vi "Application (WIP).vi"() -> ()   [LabVIEW 2018, in "Application.lvlib"]
uses:
  Application.lvlib
  Potentiostat Galvanostat Class/Controls/CV Parameters.ctl
  Potentiostat Galvanostat Class/Controls/OCV Parameters.ctl
  Potentiostat Galvanostat Class/Controls/CA Parameters.ctl
  Potentiostat Galvanostat Class/Controls/CP Parameters.ctl
  Potentiostat Galvanostat Class/Controls/PEIS Parameters.ctl
  Potentiostat Galvanostat Class/Controls/GEIS Parameters.ctl
  Potentiostat Galvanostat Class/Potentiostat Galvanostat.lvclass
panel:
  in  "DLL Path":path=path "C:/EC-Lab Development Package/EC-Lab Development Package/EClib.dll"
  out "Connected?":bool
  in  "Timeout":dbl=5.0 format="%#_g s"
  in  "IP Address/USB":string="192.109.209.128"
  in  "Disconnect":bool
  in  "Connect":bool
  out "Number of Connected PCs":i32
  out "Number of Slots":i32
  out "Number of Channels":i32
  out "Firmware Date":string
  out "Firmware Version":i32
  out "Device Code":string
  in  "Graph":bool
  in  "Stop":bool
  in  "Start":bool
  in  "Technique Parameters Tab":enum32{"ocv", "cv", "ca", "cp", "peis", "geis"}(tab)=enum."cv" caption="Parameters"
  in  "OCV Parameters":T1={"Rest duration (s)"=1.0, "Record every dE (V)"=0.01, "Record every dT (s)"=0.01, "Ewe range"=3, "CE to ground Mode"=0} {"Ewe range" items=["±2.5V", "±5V", "±10V", "Auto"]; "Record every dT (s)" min=0 format="%.2e"; "Record every dE (V)" min=0 max=100 format="%.4f"; "Rest duration (s)" min=0 format="%.2f"; "CE to ground Mode" items=["Standard", "CE to ground"]}
  in  "CV Parameters":T2={"Ei Params"={"Current step vs initial one (Ei)"=TRUE, "Voltage step (V) (Ei)"=0.0, "slew rate array (mV/s) (Ei)"=0.1}, "E1 Params"={"Current step vs initial one (E1)"=FALSE, "Voltage step (V) (E1)"=0.1, "slew rate array (mV/s) (E1)"=0.1}, "E2 Params"={"Current step vs initial one (E2)"=FALSE, "Voltage step (V) (E2)"=-0.2, "slew rate array (mV/s) (E2)"=0.1}, "Ef Params"={"Current step vs initial one (Ef)"=TRUE, "Voltage step (V) (Ef)"=0.0, "slew rate array (mV/s) (Ef)"=0.1}, "Number of cycle"=1, "recording on dE (V)"=0.01, "average every dE"=TRUE, "Begin step accumulation (1 = 100% of step)"=0.5, "End step accumulation ( 1 = 100% of step)"=0.75, "I range"=12, "Bandwidth"=5, "Ewe range"=3, "CE to ground Mode"=0} {"CE to ground Mode" items=["Standard", "CE to ground"]; "Ewe range" items=["±2.5V", "±5V", "±10V", "Auto"]; "Bandwidth" items=["1 - slow"=1, "2"=2, "3"=3, "4"=4, "5 - medium"=5, "6"=6, "7 - fast"=7]; "I range" items=["1pA", "1nA", "10nA", "100nA", "1µA", "10µA", "100µA", "1mA", "10mA", "100mA", "1A", "Booster", "Auto"]; "End step accumulation ( 1 = 100% of step)" min=0 max=1 format="%_2f"; "Begin step accumulation (1 = 100% of step)" min=0 max=1 format="%_2f"; "recording on dE (V)" min=0 max=100 format="%^_3e"; "Number of cycle" min=0 max=1000000; "Ef Params"."slew rate array (mV/s) (Ef)" min=1e-07 max=100000 format="%_5e"; "Ef Params"."Voltage step (V) (Ef)" min=-10 max=10 format="%_5e"; "E2 Params"."slew rate array (mV/s) (E2)" min=1e-07 max=100000 format="%_5e"; "E2 Params"."Voltage step (V) (E2)" min=-10 max=10 format="%_5e"; "E1 Params"."slew rate array (mV/s) (E1)" min=1e-07 max=100000 format="%_5e"; "E1 Params"."Voltage step (V) (E1)" min=-10 max=10 format="%_5e"; "Ei Params"."slew rate array (mV/s) (Ei)" min=1e-07 max=100000 format="%_5e"; "Ei Params"."Voltage step (V) (Ei)" min=-10 max=10 format="%_5e"}
  in  "CA Parameters":T3={"Voltage Steps"=[{"Voltage step vs initial one"=TRUE, "Voltage step (V)"=0.0, "Duration step (s)"=1.0}, {"Voltage step vs initial one"=TRUE, "Voltage step (V)"=0.1, "Duration step (s)"=1.0}, {"Voltage step vs initial one"=TRUE, "Voltage step (V)"=0.2, "Duration step (s)"=1.0}], "No. of steps"=2, "Record every dt (s)"=0.01, "Record every dI (A)"=1e-05, "No. of times\ntechnique is repeated"=0, "I range"=12, "Ewe range"=3, "Bandwidth"=5, "CE to ground Mode"=0} {"Voltage Steps"."Duration step (s)" min=0.001 max=80000 format="%^_3e"; "Voltage Steps"."Voltage step (V)" min=-10 max=10 format="%^_3e"; "No. of times\ntechnique is repeated" min=0 max=1000000; "No. of steps" min=0 max=99; "Record every dt (s)" min=0.0001 max=1000 format="%^_3e"; "Record every dI (A)" format="%^_3e"; "CE to ground Mode" items=["Standard", "CE to ground"]; "Ewe range" items=["±2.5V", "±5V", "±10V", "Auto"]; "Bandwidth" items=["1 - slow"=1, "2"=2, "3"=3, "4"=4, "5 - medium"=5, "6"=6, "7 - fast"=7]; "I range" items=["1pA", "1nA", "10nA", "100nA", "1µA", "10µA", "100µA", "1mA", "10mA", "100mA", "1A", "Booster", "Auto"]}
  in  "CP Parameters":T4={"Current Steps"=[{"Current step vs initial\none"=FALSE, "Current step (A)"=0.0, "Duration step (s)"=1.0}, {"Current step vs initial\none"=FALSE, "Current step (A)"=0.001, "Duration step (s)"=1.0}, {"Current step vs initial\none"=FALSE, "Current step (A)"=0.005, "Duration step (s)"=1.0}], "No. of steps"=2, "Record every dt (s)"=0.05, "Record every dE (V)"=0.005, "No. of times\ntechnique is repeated"=0, "I range"=8, "Ewe range"=3, "Bandwidth"=5, "CE to ground Mode"=0} {"Current Steps"."Duration step (s)" min=0.001 max=80000 format="%^_3e"; "Current Steps"."Current step (A)" min=-150 max=150 format="%^_3e"; "No. of times\ntechnique is repeated" min=0 max=1000000; "No. of steps" min=0 max=99; "Record every dt (s)" min=0.0001 max=1000 format="%^_3e"; "Record every dE (V)" format="%^_3e"; "CE to ground Mode" items=["Standard", "CE to ground"]; "Ewe range" items=["±2.5V", "±5V", "±10V", "Auto"]; "Bandwidth" items=["1 - slow"=1, "2"=2, "3"=3, "4"=4, "5 - medium"=5, "6"=6, "7 - fast"=7]; "I range" items=["1pA", "1nA", "10nA", "100nA", "1µA", "10µA", "100µA", "1mA", "10mA", "100mA", "1A", "Booster", "Auto"]}
  in  "PEIS Parameters":T5={"Step duration (s)"=1.0, "Record every dI (A)"=0.1, "Record every dt (s)"=0.1, "Initial voltage step (V)"=0.0, "Voltage step vs initial one"=TRUE, "Initial frequency (Hz)"=100000.0, "sweep linear/logarithmic"=FALSE, "Number of frequencies"=51, "Final frequency (Hz)"=1.0, "Sine amplitude (V)"=0.01, "No. of repeat times"=1, "No. of period to wait\nbefore each frequency"=2.0, "Non-stationary correction"=TRUE, "I Range"=12, "Bandwidth"=5, "CE to ground Mode"=0} {"CE to ground Mode" items=["Standard", "CE to ground"]; "Bandwidth" items=["1 - slow"=1, "2"=2, "3"=3, "4"=4, "5 - medium"=5, "6"=6, "7 - fast"=7]; "I Range" items=["1pA", "1nA", "10nA", "100nA", "1µA", "10µA", "100µA", "1mA", "10mA", "100mA", "1A", "Booster", "Auto"]; "No. of period to wait\nbefore each frequency" min=0 format="%.2f"; "No. of repeat times" min=1 max=1000 step=1; "Sine amplitude (V)" min=0.0005 max=0.5 format="%.2e"; "Final frequency (Hz)" min=1e-05 max=1000000 format="%.2e"; "Number of frequencies" min=1 max=10000; "Initial frequency (Hz)" min=1e-05 max=1000000 format="%.2e"; "Initial voltage step (V)" min=-10 max=10 format="%.5f"; "Record every dt (s)" min=0 format="%.2e"; "Record every dI (A)" min=0 format="%.2e"; "Step duration (s)" min=0 format="%.5f"}
  in  "GEIS Parameters":T6={"Initial frequency (Hz)"=100000.0, "sweep linear/logarithmic"=FALSE, "Number of frequencies"=51, "Final frequency (Hz)"=1.0, "Sine amplitude (A)"=0.001, "No. of repeat times"=1, "No. of period to wait\nbefore each frequency"=2.0, "Non-stationary correction"=TRUE, "I Range"=7, "Bandwidth"=5, "CE to ground Mode"=0, "Step duration (s)"=1.0, "Record every dE (V)"=0.1, "Record every dt (s)"=0.1, "Initial current step (A)"=0.0, "Current step vs initial one"=TRUE} {"Initial current step (A)" min=-10 max=10 format="%.5f"; "Record every dt (s)" min=0 format="%.2e"; "Record every dE (V)" min=0 format="%.2e"; "Step duration (s)" min=0 format="%.5f"; "CE to ground Mode" items=["Standard", "CE to ground"]; "Bandwidth" items=["1 - slow"=1, "2"=2, "3"=3, "4"=4, "5 - medium"=5, "6"=6, "7 - fast"=7]; "I Range" items=["1pA", "1nA", "10nA", "100nA", "1µA", "10µA", "100µA", "1mA", "10mA", "100mA", "1A", "Booster", "Auto"]; "No. of period to wait\nbefore each frequency" min=0 format="%.2f"; "No. of repeat times" min=1 max=1000 step=1; "Sine amplitude (A)" min=0 max=100 format="%.2e"; "Final frequency (Hz)" min=1e-05 max=1000000 format="%.2e"; "Number of frequencies" min=1 max=10000; "Initial frequency (Hz)" min=1e-05 max=1000000 format="%.2e"}
  in  "Technique":T7(ring)=enum."Cyclic Voltammetry"
  out "Channel Information":T8
  in  "Plugged Channels":string(combo)
  in  "Table Tab":enum32{"Process 0", "Process 1"}(tab)
  out "Process 0 Table":string[][](table)
  out "Process 1 Table":string[][](table)
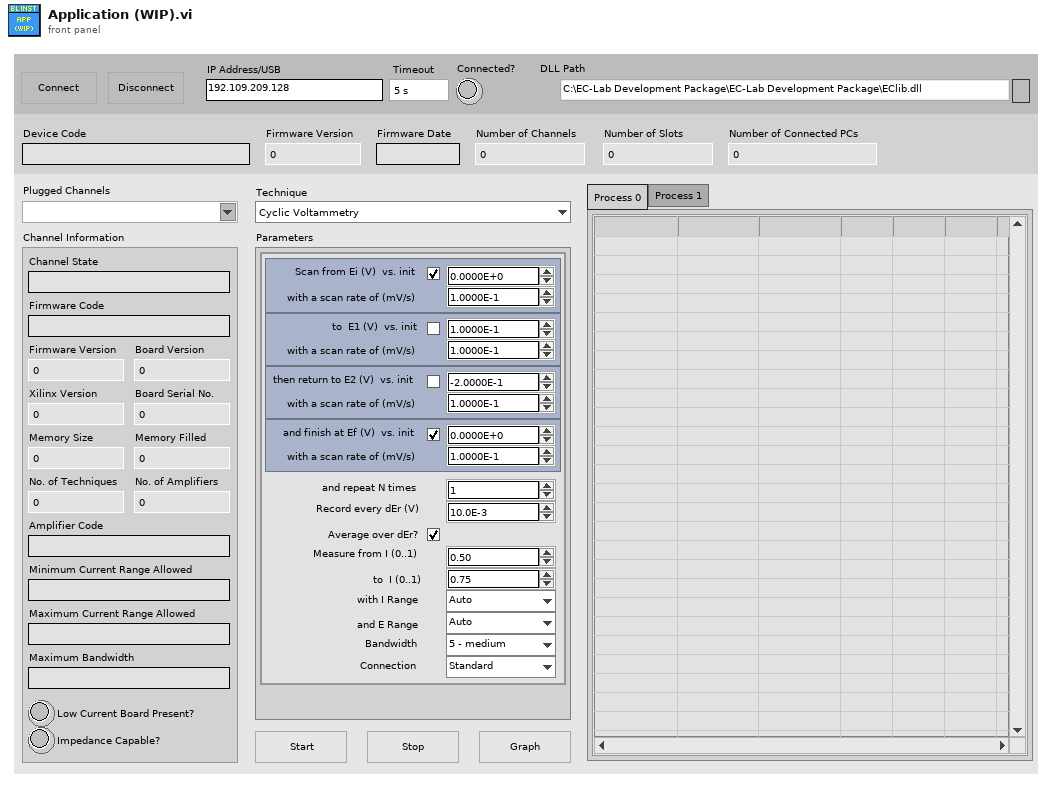
[diagram p1: front panel]
types:
  T1 = typedef "Potentiostat Galvanostat.lvclass/OCV Parameters.ctl" = cluster{"Rest duration (s)":sgl, "Record every dE (V)":sgl, "Record every dT (s)":sgl, "Ewe range":u16, "CE to ground Mode":u16}
  T2 = typedef "Potentiostat Galvanostat.lvclass/CV Parameters.ctl" = cluster{"Ei Params":cluster{"Current step vs initial one (Ei)":bool, "Voltage step (V) (Ei)":sgl, "slew rate array (mV/s) (Ei)":sgl}, "E1 Params":cluster{"Current step vs initial one (E1)":bool, "Voltage step (V) (E1)":sgl, "slew rate array (mV/s) (E1)":sgl}, "E2 Params":cluster{"Current step vs initial one (E2)":bool, "Voltage step (V) (E2)":sgl, "slew rate array (mV/s) (E2)":sgl}, "Ef Params":cluster{"Current step vs initial one (Ef)":bool, "Voltage step (V) (Ef)":sgl, "slew rate array (mV/s) (Ef)":sgl}, "Number of cycle":i32, "recording on dE (V)":sgl, "average every dE":bool, "Begin step accumulation (1 = 100% of step)":sgl, "End step accumulation ( 1 = 100% of step)":sgl, "I range":u16, "Bandwidth":u16, "Ewe range":u16, "CE to ground Mode":u16}
  T3 = typedef "Potentiostat Galvanostat.lvclass/CA Parameters.ctl" = cluster{"Voltage Steps":cluster{"Voltage step vs initial one":bool, "Voltage step (V)":sgl, "Duration step (s)":sgl}[], "No. of steps":i32, "Record every dt (s)":sgl, "Record every dI (A)":sgl, "No. of times\ntechnique is repeated":i32, "I range":u16, "Ewe range":u16, "Bandwidth":u16, "CE to ground Mode":u16}
  T4 = typedef "Potentiostat Galvanostat.lvclass/CP Parameters.ctl" = cluster{"Current Steps":cluster{"Current step vs initial\none":bool, "Current step (A)":sgl, "Duration step (s)":sgl}[], "No. of steps":i32, "Record every dt (s)":sgl, "Record every dE (V)":sgl, "No. of times\ntechnique is repeated":i32, "I range":u16, "Ewe range":u16, "Bandwidth":u16, "CE to ground Mode":u16}
  T5 = typedef "Potentiostat Galvanostat.lvclass/PEIS Parameters.ctl" = cluster{"Step duration (s)":sgl, "Record every dI (A)":sgl, "Record every dt (s)":sgl, "Initial voltage step (V)":sgl, "Voltage step vs initial one":bool, "Initial frequency (Hz)":sgl, "sweep linear/logarithmic":bool, "Number of frequencies":i32, "Final frequency (Hz)":sgl, "Sine amplitude (V)":sgl, "No. of repeat times":i32, "No. of period to wait\nbefore each frequency":sgl, "Non-stationary correction":bool, "I Range":u16, "Bandwidth":u16, "CE to ground Mode":u16}
  T6 = typedef "Potentiostat Galvanostat.lvclass/GEIS Parameters.ctl" = cluster{"Initial frequency (Hz)":sgl, "sweep linear/logarithmic":bool, "Number of frequencies":i32, "Final frequency (Hz)":sgl, "Sine amplitude (A)":sgl, "No. of repeat times":i32, "No. of period to wait\nbefore each frequency":sgl, "Non-stationary correction":bool, "I Range":u16, "Bandwidth":u16, "CE to ground Mode":u16, "Step duration (s)":sgl, "Record every dE (V)":sgl, "Record every dt (s)":sgl, "Initial current step (A)":sgl, "Current step vs initial one":bool}
  T7 = enum16{"Open Circuit Voltage", "Cyclic Voltammetry", "Chrono-Amperometry", "Chrono-Potentiometry", "Potentio Electrochemical Impedance Spectroscopy", "Galvano Electrochemical Impedance Spectroscopy"}
  T8 = cluster{"Firmware Code":string, "Firmware Version":i32, "Board Version":i32, "Channel State":string, "Board Serial No.":i32, "Xilinx Version":i32, "Memory Size":i32, "Memory Filled":i32, "No. of Techniques":i32, "No. of Amplifiers":i32, "Amplifier Code":string, "Minimum Current Range Allowed":string, "Maximum Current Range Allowed":string, "Maximum Bandwidth":string, "Impedance Capable?":bool, "Low Current Board Present?":bool}
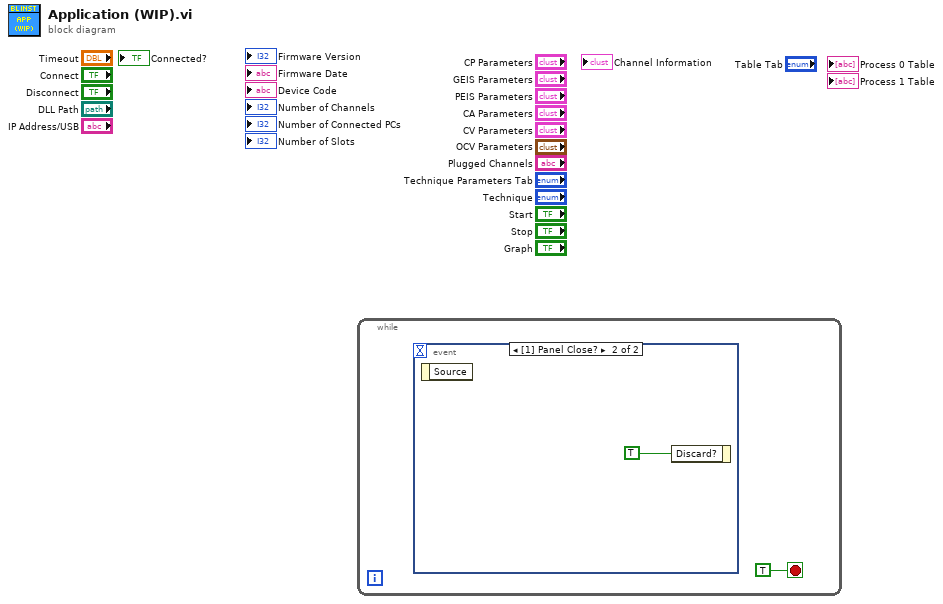
[diagram p0: block diagram]
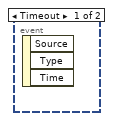
[diagram p2: hidden frame]
diagram:
  n1 = while {
    stop <- TRUE stop-if-true
    n2 = event shown="[1] Panel Close?" {
      selector: _ -> [_ _]
      dyn-events: _ -> [_ _]
      timeout: _ -> [_ _]
      event Timeout {
        n3 = event-data() -> ()  [unwired: 1 in, 3 out]
      }
      event Panel Close? {
        n4 = event-data() -> ()  [unwired: 1 in, 1 out]
        n5 = event-data("Discard?"=TRUE) -> ()  [unwired: 1 in, 1 out]
      }
    }
  }
